vi "Write Panel Bounds.vi"(5 "Panel Bounds":T1, 9 "FPWindow in":refnum<class "FPWindow.lvclass">) -> (3 "FPWindow out":refnum<class "FPWindow.lvclass">)   [LabVIEW 2014, in "FPWindow.lvclass"]
uses:
  FPWindow.lvclass
  <vilib>/Utility/miscctls.llb/LVRectTypeDef.ctl
  FPWindow.lvclass/FPWindow.ctl
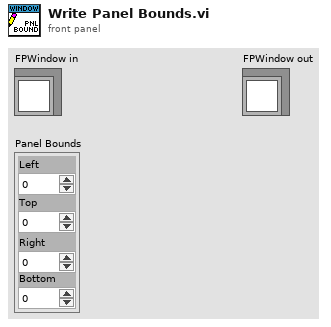
[diagram p1: front panel]
types:
  T1 = typedef "LVRectTypeDef.ctl" = cluster{"Left":i16, "Top":i16, "Right":i16, "Bottom":i16}
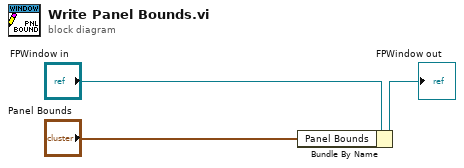
[diagram p0: block diagram]
diagram:
  n1 = Bundle By Name(cluster="FPWindow in", "Panel Bounds"="Panel Bounds") -> (→"FPWindow out":refnum<class "FPWindow.lvclass">)
